vi "De-queue RT data element.vi"(11 "RT Queues":T1) -> (0 "timed out?":bool, 1 "Data":variant, 3 "Message":string)   [LabVIEW 2018]
uses:
  Type Defs/Queues cluster.ctl
  ICL-LabVIEW_General/Message Scheduler/message scheduler.lvclass
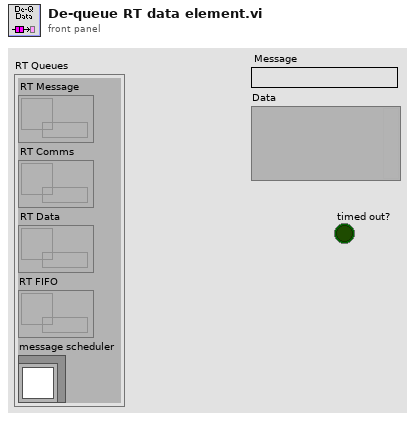
[diagram p1: front panel]
types:
  T1 = typedef "Queues cluster.ctl" = cluster{"RT Message":refnum<queue>, "RT Comms":refnum<queue>, "RT Data":refnum<queue>, "RT FIFO":refnum<queue>, "message scheduler":refnum<class "message scheduler.lvclass">}
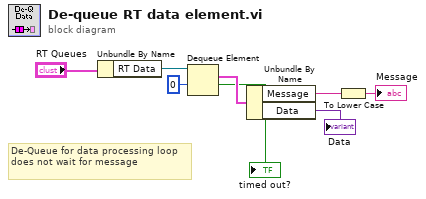
[diagram p0: block diagram]
diagram:
  # "De-Queue for data processing loop does not wait for message"
  n1 = Unbundle By Name("RT Queues") -> ("RT Data"=w7:refnum<queue>)
  n2 = Dequeue Element(queue=w7, timeout in ms (-1)=0) -> (element=w6:cluster{"Message":string, "Data":variant}, timed out?=→"timed out?":bool)  [unwired: 1 in, 2 out]
  n3 = Unbundle By Name(w6) -> ("Message"=w5:string, "Data"=→"Data":variant)
  n4 = To Lower Case(string=w5) -> (all lower case string=→"Message":string)
